vi "PathPlanner_PathFinder_ExtractPathSub1ALT.vi"(9 "SStart":T1, 10 "SGoal":T1, 11 "PathPoints In":T1[](array[typedef])) -> (3 "Path Points Out":T1[](array[typedef]))   [LabVIEW 2019, in "PathPlanner24.lvlib"]
doc: "Internal function. Not to be used by end users."
uses:
  PathPlanner24.lvlib
  TypeDef/PathPlannerFinderGridPosition.ctl
  <vilib>/robotics/Navigation/shared/MapNode/AbstractDstarNode/NI_Robotics_AbstractDstarNode.lvclass
  C:/Program Files/National Instruments/LabVIEW 2019/vi.lib/robotics/Navigation/shared/MapNode/AbstractAstarNode/NI_Robotics_AbstractAstarNode.lvclass
  PathPlanner_PathFinder_Globals.vi
  <vilib>/robotics/Navigation/shared/WorldMap/OccupancyGridWorldMap/NI_Robotics_OccupancyGridWorldMap.lvclass
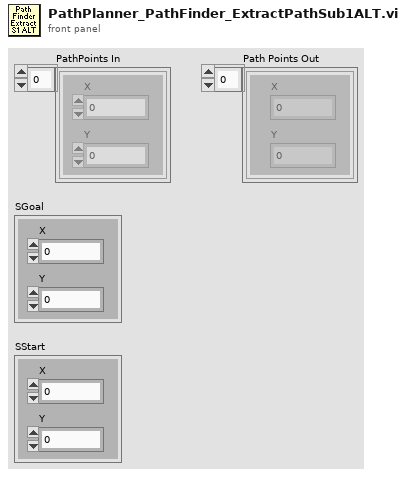
[diagram p1: front panel]
types:
  T1 = typedef "PathPlanner24.lvlib/PathPlannerFinderGridPosition.ctl" = cluster{"X":i32, "Y":i32}
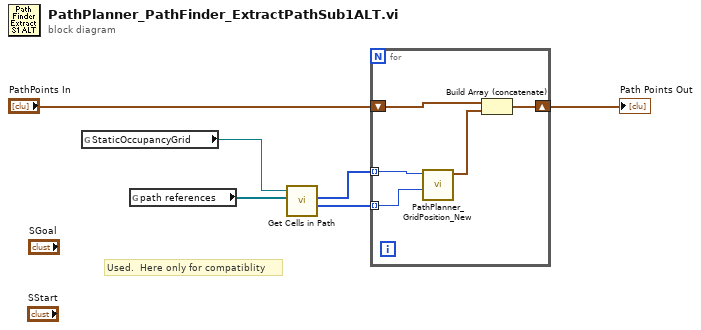
[diagram p0: block diagram]
diagram:
  # "Used.  Here only for compatiblity"
  n1 = global read "PathPlanner_PathFinder_Globals.vi" "StaticOccupancyGrid"() -> (w6:refnum<data-value>)
  n2 = global read "PathPlanner_PathFinder_Globals.vi" "path references"() -> (w5:refnum<data-value>[])
  n3 = call <vilib>:"Get Cells in Path.vi"("path references"=w5, "map reference in"=w6) -> ("y coordinates"=w3:i32[], "x coordinates"=w4:i32[])  [unwired: 6 in, 2 out]
  n4 = for {
    tunnel: w4 -> [w9] mode=indexing
    tunnel: w3 -> [w8] mode=indexing
    shift-right: [w11] -> w1
    shift-left: "PathPoints In" -> [w10]
    n5 = call "PathPlanner_GridPosition_New.vi"("Int Y"=w8, "Int X"=w9) -> ("GridPosition"=w7:T1)  [unwired: 9 in]
    n6 = Build Array (concatenate)(w10, w7) -> (w11:T1[])
  }
  "Path Points Out" <- w1
